vi "Stop Core.vi"(10 "最终错误代码":i32, 11 "蒸发冷却器":refnum<class "Evaporative Cooler.lvclass">) -> (3 "蒸发冷却器":refnum<class "Evaporative Cooler.lvclass">)   [LabVIEW 2013, in "Evaporative Cooler.lvlib" / "Evaporative Cooler.lvclass"]
doc: "对于操作者运行过程中创建的所有并行进程，在重写Stop Core.vi的VI中应调用必要代码使其停止运行。需要停止的进程包括该操作本身创建的层层嵌套的操作者，以及所有其他异步运行的VI，比如时间延迟消息。需要停止的进程可能还包括Actor Core中的所有并行循环。（另一种方法，是在Actor Core程序框图上，在“调用父节点”结束时触发一个局部信号来停止这些进程。）\n\n<b>最终错误代码</b>输入表示操作者退出时设定的错误。0表示无错误。该错误代码可用于区分“正常停止”和“紧急停止”，从而向其他操作者发送信号。一般用非零值表示“紧急停止”，当然对于某个特定的操作者也可采用其他的表示方法。请注意，1608是个特殊的错误代码，表示当前操作者本身被“紧急停止”，如出现该错误，只能直接传递该代码。"
uses:
  Evaporative Cooler.lvclass
  <vilib>/ActorFramework/Time-Delayed Send Message/Time-Delay Override Options.ctl
  Cooler/Cooler/Cooler.lvclass
  Evaporative Cooler.lvclass/Evaporative Cooler.ctl
  <vilib>/ActorFramework/Stop Msg/Stop Msg.lvclass/Stop Msg.ctl
  <vilib>/ActorFramework/Message Enqueuer/Message Enqueuer.lvclass/Message Enqueuer.ctl
  <vilib>/ActorFramework/Stop Msg/Send Emergency Stop.vi
  <vilib>/ActorFramework/Stop Msg/Send Normal Stop.vi
  <vilib>/ActorFramework/Message Enqueuer/Enqueue Critical.vi
  <vilib>/ActorFramework/Message Enqueuer/Enqueue.vi
  <vilib>/ActorFramework/Message Priority Queue/Priority Enqueue.vi
  <vilib>/ActorFramework/Stop Msg/Stop Msg.lvclass
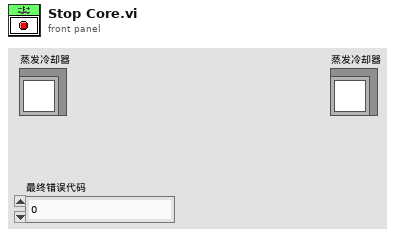
[diagram p1: front panel]
types:
  T1 = typedef "Time-Delay Override Options.ctl" = enum16{"Send next copy now", "Skip next scheduled copy", "Send next copy now and stop all further copies", "Stop all further copies"}
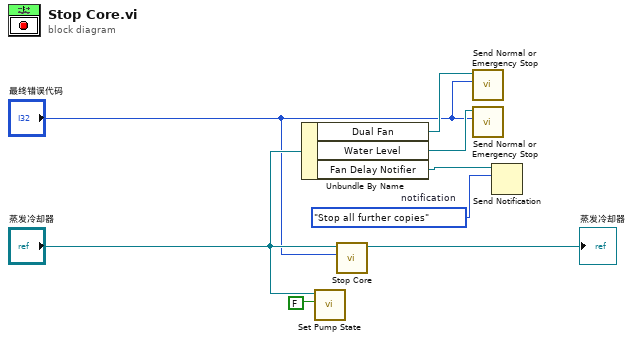
[diagram p0: block diagram]
diagram:
  w7 = Time-Delay_Override_Options."Stop all further copies"  # notification
  n1 = Unbundle By Name("蒸发冷却器") -> ("Dual Fan"=w3:refnum<class "Message Enqueuer.lvclass">, "Water Level"=w2:refnum<class "Message Enqueuer.lvclass">, "Fan Delay Notifier"=w6:refnum<notifier>)
  n2 = call-dynamic "Set Pump State.vi"("泵状态"=FALSE ("Pump State"), "蒸发冷却器输入"="蒸发冷却器") -> ()  [unwired: 9 in, 1 out]
  n3 = call-parent "Stop Core.vi"("final error code"="最终错误代码", "Actor in"="蒸发冷却器") -> ("Actor out"=→"蒸发冷却器":refnum<class "Evaporative Cooler.lvclass">)  [unwired: 9 in]
  n4 = call <vilib>:"Send Normal or Emergency Stop.vi"("final error code"="最终错误代码", "Message Enqueuer"=w3) -> ()  [unwired: 9 in, 1 out]
  n5 = call <vilib>:"Send Normal or Emergency Stop.vi"("final error code"="最终错误代码", "Message Enqueuer"=w2) -> ()  [unwired: 9 in, 1 out]
  n6 = Send Notification(notification=w7, notifier=w6) -> ()  [unwired: 1 in, 2 out]
